vi "DT_Merge_Update Candidate.vi"(10 "Data In":T1, 11 "Triangles In":i32[][](array[numeric])) -> (2 "Data Out":T1, 3 "Triangles Out":i32[][](array[numeric]))   [LabVIEW 2017, in "NI_AAL_Geometry.lvlib"]
uses:
  <vilib>/Analysis/NI_AAL_Geometry.lvlib
  <vilib>/Analysis/geometry.llb/DT_Merge_Find Next Triangulation_Data.ctl
  <vilib>/Analysis/geometry.llb/DT_Triangle Manager_Get Oppo Point_in Ghost.vi
  <vilib>/Analysis/geometry.llb/DT_Triangle Manager_Get Global Point Index.vi
  <vilib>/Analysis/geometry.llb/DT_Triangle Manager_Get Adj_by Edge.vi
  <vilib>/Analysis/geometry.llb/DT_Triangle Manager_Get Local Point Index.vi
  <vilib>/Analysis/geometry.llb/DT_Triangle Manager_Get Oppo Point.vi
  <vilib>/Analysis/geometry.llb/DT_Triangle Manager_Get Ghost Point.vi
  <vilib>/Analysis/geometry.llb/DT_Triangle Manager_Get Adj_by Point.vi
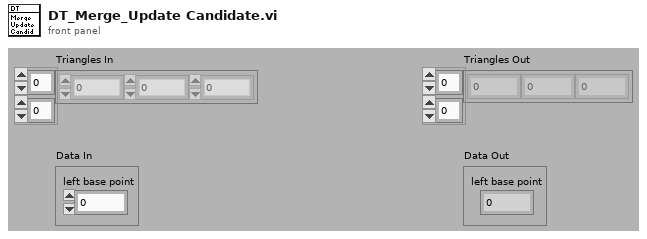
[diagram p1: front panel]
types:
  T1 = typedef "NI_AAL_Geometry.lvlib/DT_Merge_Find Next Triangulation_Data.ctl" = cluster{"left base point":i32, "left triangle":i32, "left local idx":i32, "right base point":i32, "right triangle":i32, "right local idx":i32, "Left Candidate Triangles":i32[], "Left Candidate Point Idx":i32[], "Right Candidate Triangles":i32[], "Right Candidate Point Idx":i32[], "cur triangle":i32}
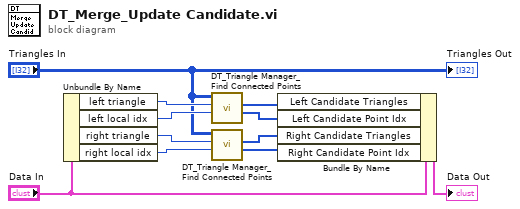
[diagram p0: block diagram]
diagram:
  n1 = Unbundle By Name("Data In") -> ("left triangle"=w11:i32, "left local idx"=w10:i32, "right triangle"=w5:i32, "right local idx"=w4:i32)
  n2 = call <vilib>:"DT_Triangle Manager_Find Connected Points.vi"("base point idx"=w10, "triangle"=w11, "Triangles"="Triangles In") -> ("Connected Point Idx"=w8:i32[], "Connected Triangles"=w9:i32[])  [unwired: 7 out]
  n3 = call <vilib>:"DT_Triangle Manager_Find Connected Points.vi"("base point idx"=w4, "triangle"=w5, "Triangles"="Triangles In") -> ("Connected Point Idx"=w2:i32[], "Connected Triangles"=w3:i32[])  [unwired: 7 out]
  n4 = Bundle By Name(cluster="Data In", "Left Candidate Triangles"=w9, "Left Candidate Point Idx"=w8, "Right Candidate Triangles"=w3, "Right Candidate Point Idx"=w2) -> (→"Data Out":T1)
  "Triangles Out" <- "Triangles In"
